vi "GenerateLogFile.vi"(7 "Mixture Strings":string[](array[string]), 8 "Sequence Time":dbl[](array[numeric]), 9 "Mix Sequence Array":bool[][](array[boolean]), 10 "Concentration Names":string[](array[string]), 11 "Odor Names":string[](array[string])) -> (1 "Log Cluster":T1, 3 "Text Log Data":string[][](array[string]))   [LabVIEW 2016]
panel:
  out "Array":string[](array[string])
  out "lines":string[](array[string])
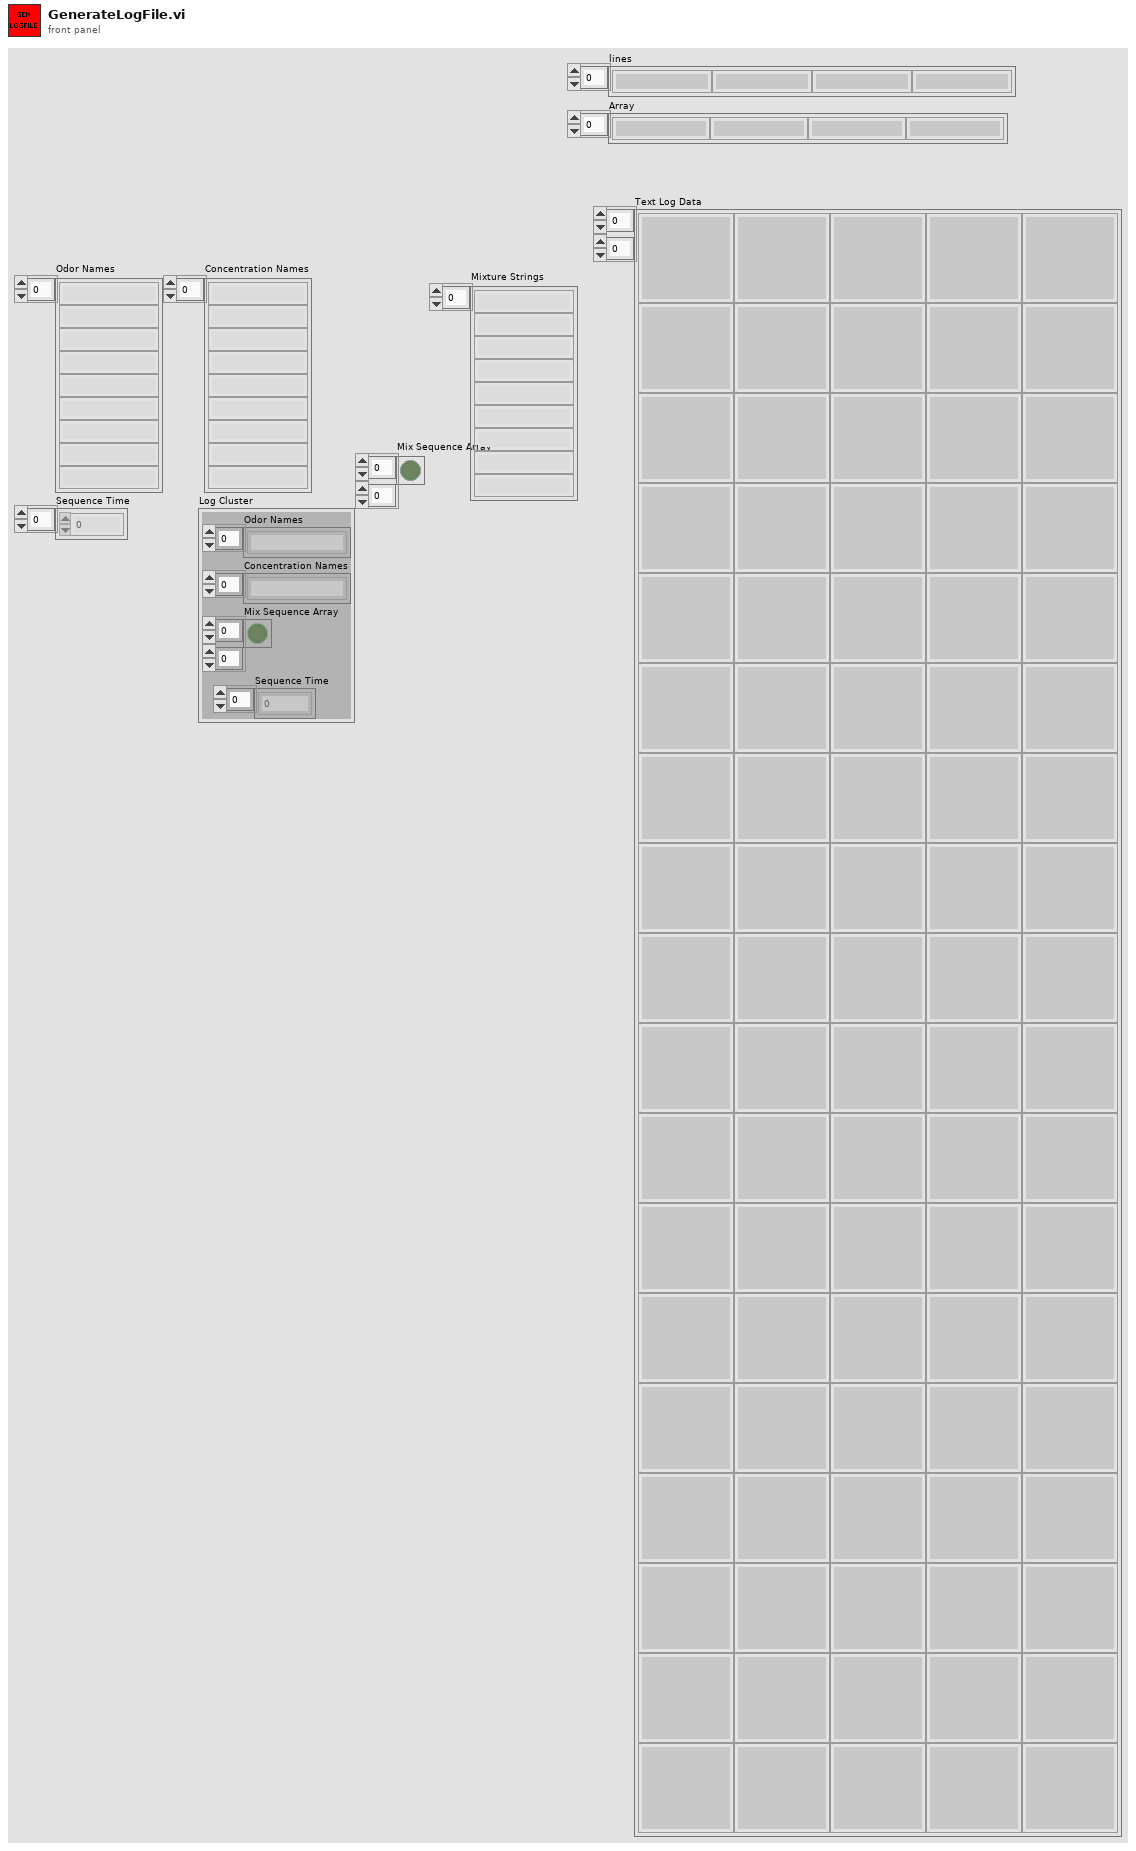
[diagram p1: front panel]
types:
  T1 = cluster{"Odor Names":string[], "Concentration Names":string[], "Mix Sequence Array":bool[][], "Sequence Time":dbl[]}
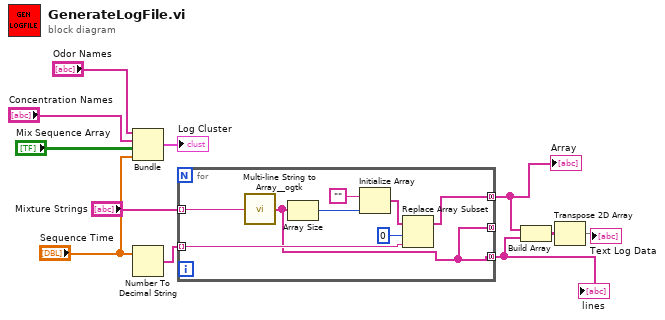
[diagram p0: block diagram]
diagram:
  n1 = Bundle("Odor Names"="Odor Names", "Concentration Names"="Concentration Names", "Mix Sequence Array"="Mix Sequence Array", "Sequence Time"="Sequence Time") -> (→"Log Cluster":T1)  [unwired: 1 in]
  n2 = Number To Decimal String(number="Sequence Time") -> (decimal integer string=w5:string[])  [unwired: 1 in]
  n3 = for {
    tunnel: "Mixture Strings" -> [w19] mode=indexing
    tunnel: w5 -> [w14] mode=indexing
    tunnel: [w12] -> _ mode=concatenating
    tunnel: [w12] -> w3 mode=concatenating
    tunnel: [w13] -> w4 mode=concatenating
    n4 = call <userlib>:"Multi-line String to Array__ogtk.vi"("string"=w19) -> ("lines"=w12:string[])
    n5 = Array Size(array=w12) -> (size(s)=w18:i32)
    n6 = Initialize Array("", w18) -> (w16:string[])
    n7 = Replace Array Subset(array=w16, new element=w14, index=0) -> (w13:string[])
  }
  "lines" <- w3
  "Array" <- w4
  n8 = Build Array(w4, w3) -> (w2:string[][])
  n9 = Transpose 2D Array(2D array=w2) -> (transposed array=→"Text Log Data":string[][])
